vi "Make MSB 1.vi"(11 "Register Address":u8) -> (3 "Register Address | 0x80":u8)   [LabVIEW 2020, in "LINX I2C.lvclass"]
doc: "Makes the MSB of the byte a 1 by ORing with 0x80 - used for enabling auto-increment on I2C register reads. Only functions for U8s."
uses:
  LINX I2C.lvclass
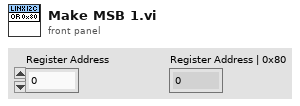
[diagram p1: front panel]
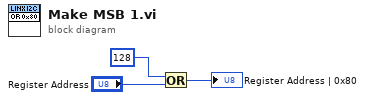
[diagram p0: block diagram]
diagram:
  n1 = Or(x=u8 128, y="Register Address") -> (x .or. y?=→"Register Address | 0x80":u8)
